vi "MPS_Spectroscopy_Core.vi"(0 "EmptyBoreBaseline_Spec":dbl[](array[numeric])=array[21000 elements], 1 "ms delay":u32=25 format="%#.4p", 3 "Spec samples\nto crop":dbl=1000.0 format="%#_4p") -> (5 "Raw Measured":dbl[](array[numeric]), 6 "f0 Complex":cdb=-0.004151438219837607-0.0046789149193528995i, 7 "phase f1-f9":dbl[](array[numeric])=[-2.296530890286755, -0.4996795442572583, 2.13231335701235, -2.8305146270300687, -3.0644603787657894, -1.910517808964867, -1.4604887262767599, -1.4608770943170013, -0.49288277337997893] format="%#_4g", 8 "TF Corr Rx FFT complex":T2, 9 "TF units from loaded file":string, 10 "Spec Waveform Baseline Sub":waveform(dbl)={"t0"=timestamp(3728232981.5205336 s since 1904-01-01), "dt"=9.9999999999997e-07, "Y"=array[20000 elements], "attributes"=variant("NI_ChannelName"=variant(string "H1/ai7"), "NI_UnitDescription"=variant(string "Volts"))}, 11 "TxIMon cluster":T1, 12 "3f0 Complex":cdb=-1.808865307320394e-10+2.875482942470047e-10i, 13 "mag f1-f9":dbl[](array[numeric])=[0.006255132621749245, 5.349180742819057e-10, 3.3971158138137566e-10, 2.020645150662673e-11, 3.443682420408273e-11, 3.747219651257019e-11, 4.2635827797213496e-11, 3.5893791114801e-11, 3.560739858812373e-11] format="%#_4p", 14 "RX magnitude 3":dbl=3.3971158138137566e-10, 15 "Expected mT Spec Drive":dbl=0.03824103018872398 format="%#_4p", 16 "TF Corrected\nMagnetization over time":waveform(dbl)[](graph), 17 "Spec Time Domain":dbl[][](graph), 18 "Amps Drive Spec":dbl=0.058832354136498434 format="%#_4p", 19 "THD":dbl=1.5484776612982656 format="%#_6p")   [LabVIEW 2021]
uses:
  <vilib>/Analysis/4window.llb/windowTd.ctl
  <extravilib>/ChannelInstances/Tag-dbl/Write With Abort.vi
  MPS_global_variables.vi
  <extravilib>/ChannelInstances/Tag-dbl/Instantiate.vi
  <extravilib>/ChannelInstances/Tag-dbl/Endpoint.vi
  <extravilib>/ChannelInstances/Tag-dbl.lvlib
  <vilib>/measure/NI_MAPro.lvlib
  <vilib>/Analysis/NI_AALPro.lvlib
  <vilib>/measure/matone.llb/Extract Single Tone Information 1 Chan.vi
  <vilib>/measure/maspectr.llb/FFT Spectrum (Mag-Phase) for 1 Chan.vi
panel:
  out "error?":bool
  out "error out":errorcluster
  out "THD dB":dbl
  out "Rx FFT _NoCorrect":cluster{"f0":dbl, "df":dbl, "magnitude":dbl[]}(graph)
  out "f0 over time 2":dbl(graph)=3.3971158138137566e-10
  out "Waveform Graph":cluster{"f0":dbl, "df":dbl, "magnitude":dbl[]}(graph)
  out "dMdt":dbl[](graph)
  out "3f0 over time":dbl(graph)=3.3971158138137566e-10
  out "Drive IMon FFT":cluster{"f0":dbl, "df":dbl, "magnitude":dbl[]}(graph)={"f0"=0.0, "df"=47.61904761904904, "magnitude"=array[10500 elements]}
  out "Drive IMon":waveform(dbl)(graph)={"t0"=timestamp(3728232981.5496345 s since 1904-01-01), "dt"=9.9999999999997e-07, "Y"=array[21000 elements], "attributes"=variant("NI_ChannelName"=variant(string "H1/ai4"), "NI_UnitDescription"=variant(string "Volts"))}
  out "detected amplitude\nDrive IMon":dbl=0.0003328133743989285 format="%.4p"
  out "Samples Per Acquisition":dbl=21000.0
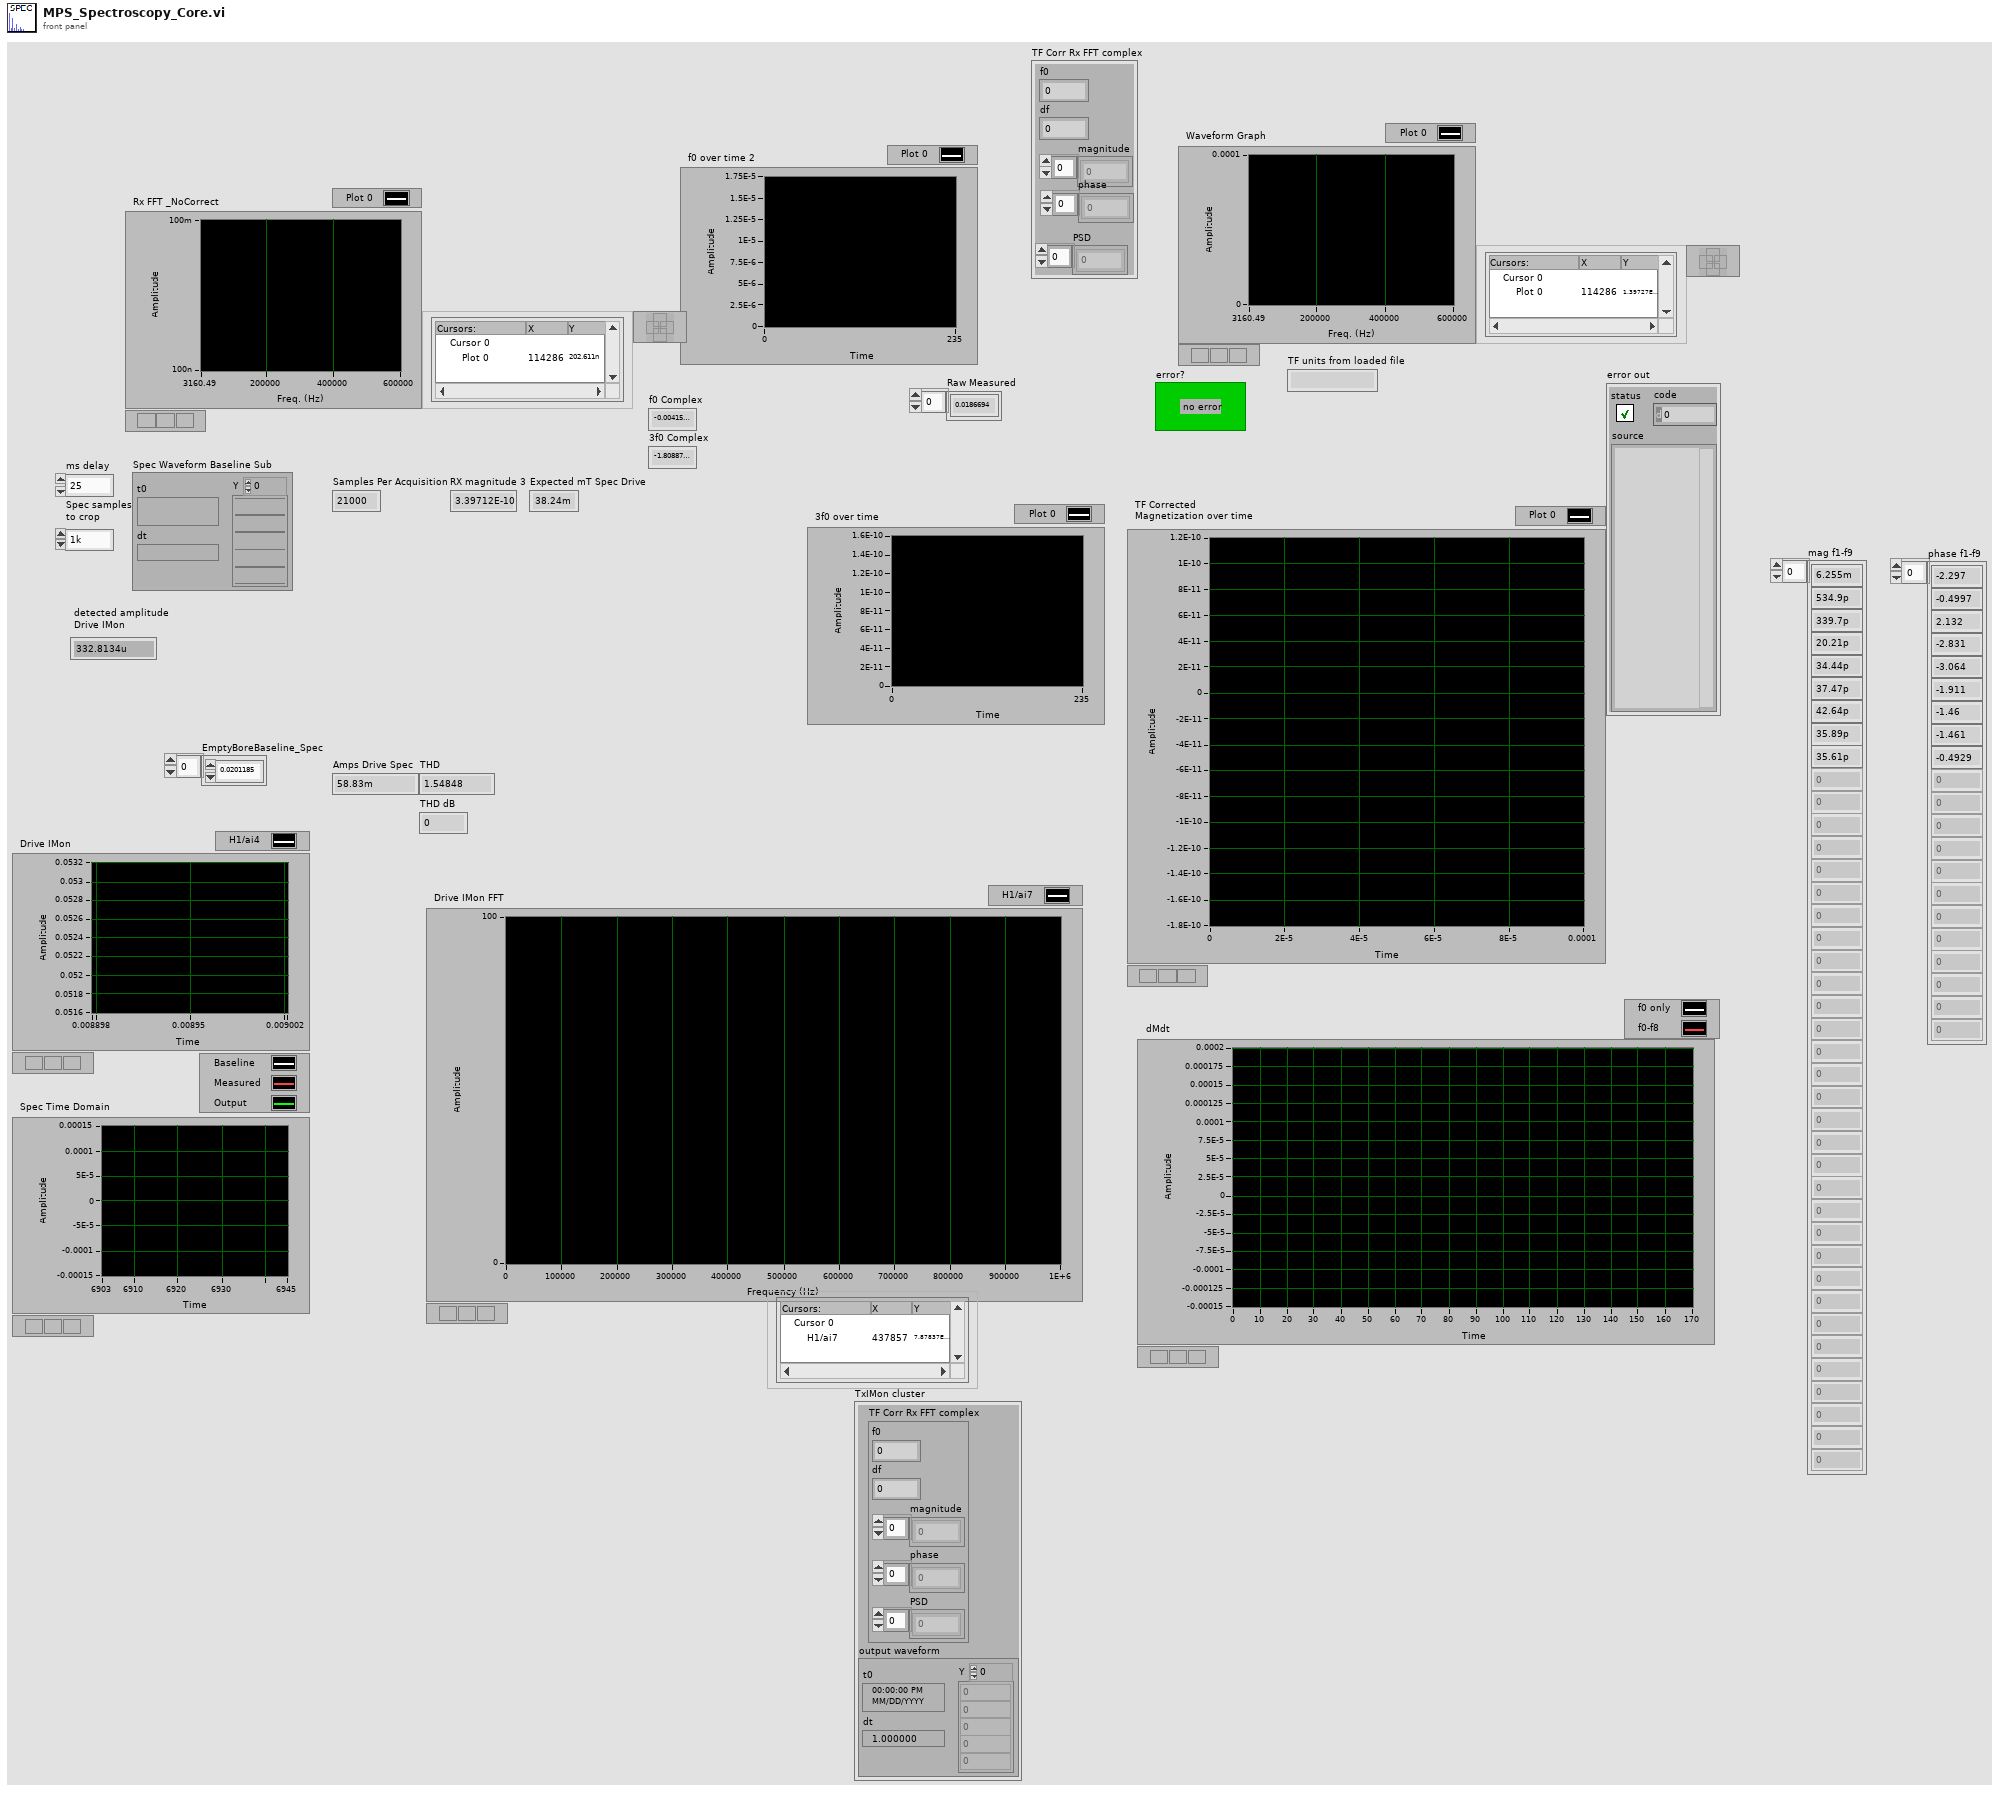
[diagram p1: front panel]
types:
  T1 = cluster{"TF Corr Rx FFT complex":cluster{"f0":dbl, "df":dbl, "magnitude":dbl[], "phase":dbl[], "PSD":dbl[]}, "output waveform":waveform(dbl)}
  T2 = cluster{"f0":dbl, "df":dbl, "magnitude":dbl[], "phase":dbl[], "PSD":dbl[]}
  T3 = cluster{"sample rate":dbl, "Transmit frequency":dbl, "Transmit amplitude":dbl, "sample rate digital out":dbl, "TX cycles":i32, "sample rate DAQ1":dbl, "Receive frequency":dbl, "Receive range":dbl, "TX harmonics":dbl[]}
  T4 = typedef "NI_AALPro.lvlib/windowTd.ctl" = u32
  T5 = cluster{"sample rate":dbl, "Tx freq":dbl, "Tx amp":dbl, "Tx cycles\nSpectroscopy":dbl, "Bias amp":dbl, "Bias freq":dbl, "Receive range":dbl, "Bias Periods\nMagnetometry":dbl, "Tx Freq Division Factor":dbl, "Drive Periods per Bias":dbl, "TX harmonics":dbl[]}
  T6 = typedef "Tag-dbl.lvlib/))Channel.ctl" = refnum<queue>
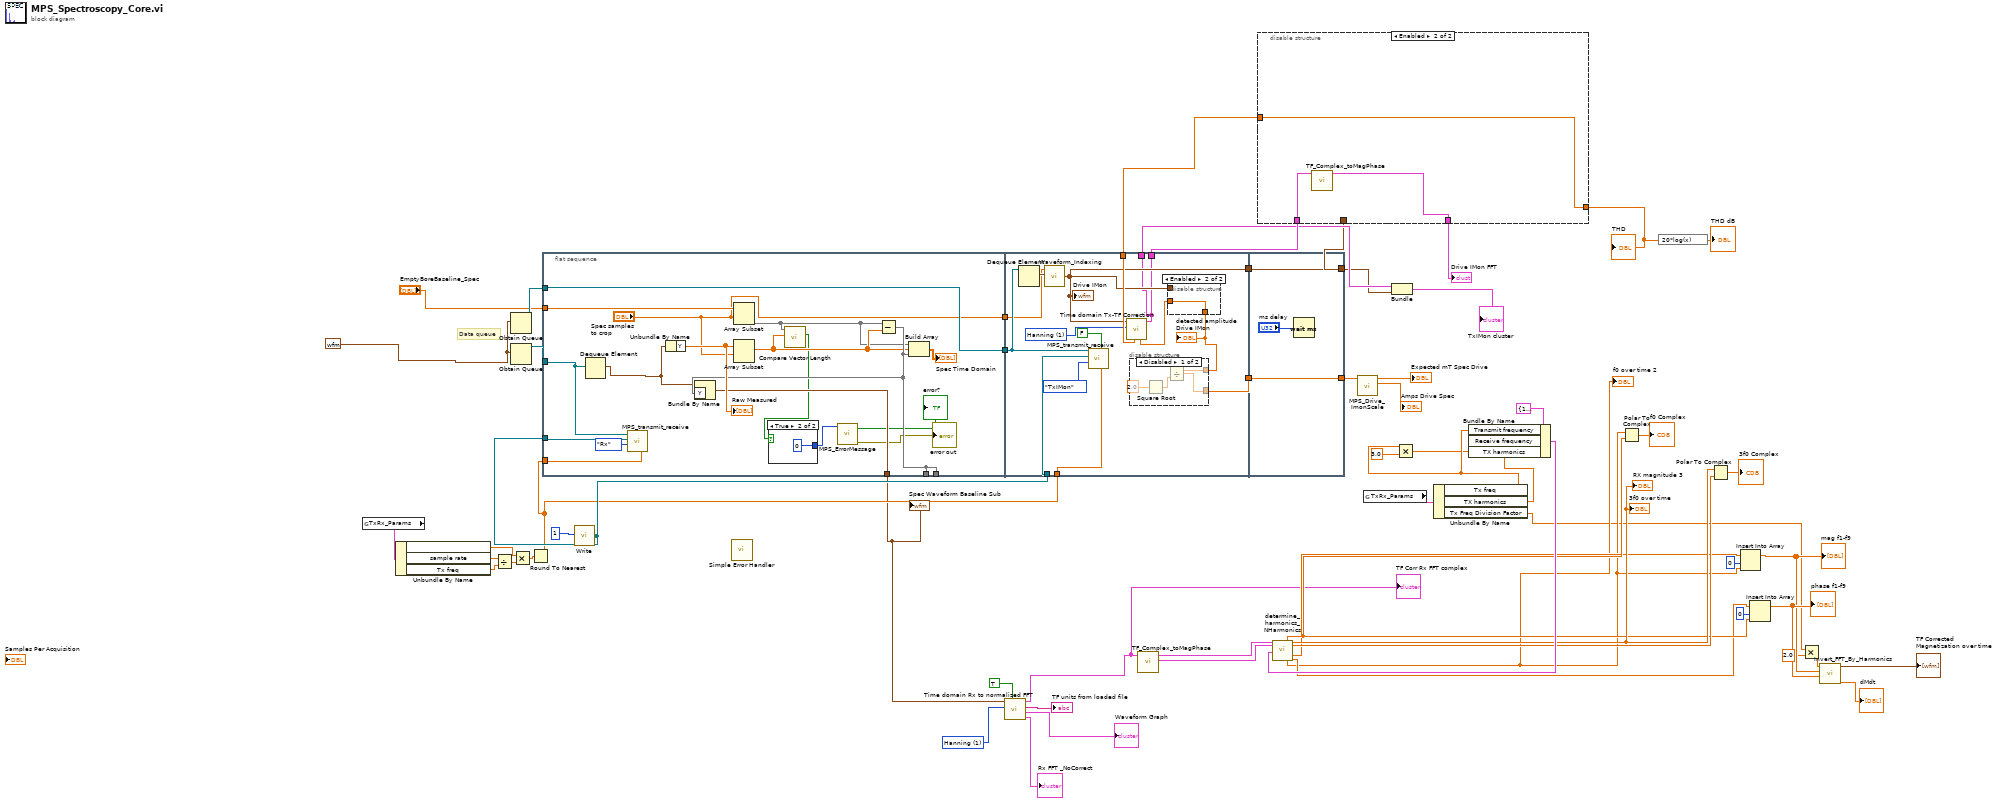
[diagram p0: block diagram]
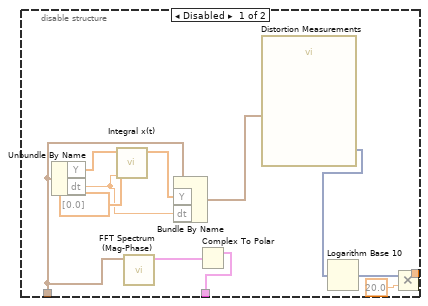
[diagram p2: hidden frame]
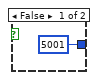
[diagram p3: hidden frame]
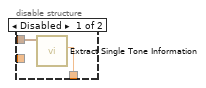
[diagram p5: hidden frame]
diagram:
  w11 = T4 1 items=["Rectangle"=0, "Hanning"=1, "Hamming"=2, "Blackman-Harris"=3, "Exact Blackman"=4, "Blackman"=5, "Flat Top"=6, "4 Term B-Harris "=7, "7 Term B-Harris"=8, "Low Sidelobe"=9, "Blackman Nuttall"=11, "Triangle"=30, "Bartlett-Hanning"=31, "Bohman"=32, "Parzen"=33, "Welch"=34, "Kaiser"=60, "Dolph-Chebyshev"=61, "Gaussian"=62] ("window")
  w23 = waveform(dbl) {"t0"=timestamp(0 s since 1904-01-01), "dt"=1.0, "Y"=[]} ("Waveform")
  # "Data queue"
  n1 = global read "MPS_global_variables.vi" "TxRx_Params"() -> (w54:T5)
  n2 = Unbundle By Name(w54) -> ("Tx cycles\nSpectroscopy"=w50:dbl, "sample rate"=w53:dbl, "Tx freq"=w52:dbl)
  n3 = Divide(x=w53, y=w52) -> (x/y=w51:dbl)
  n4 = Obtain Queue(element data type=w23) -> (queue out=w55:refnum<queue>)  [unwired: 4 in, 2 out]
  n5 = Obtain Queue(element data type=w23) -> (queue out=w56:refnum<queue>)  [unwired: 4 in, 2 out]
  n6 = Multiply(x=w50, y=w51) -> (x*y=w49:dbl)
  n7 = Round To Nearest(number=w49) -> (nearest integer value=w48:dbl)
  n8 = flat-sequence {
    tunnel: w56 -> [w78]
    tunnel: [w77] -> w61
    tunnel: w57 -> [w79]
    tunnel: w55 -> [w77]
    tunnel: w48 -> [w76]
    tunnel: [w73] -> w18
    tunnel: [w72] -> _
    tunnel: [w72] -> _
    tunnel: "EmptyBoreBaseline_Spec" -> [w71]
    tunnel: ["Spec samples\nto crop"] -> w7
    tunnel: w61 -> [w93]
    tunnel: w57 -> [w95]
    tunnel: w48 -> [w94]
    tunnel: [w84] -> w60
    tunnel: [w89] -> w59
    tunnel: [w83] -> w9
    tunnel: [w87] -> w8
    tunnel: w7 -> [w85]
    tunnel: [w83] -> w6
    tunnel: [w106] -> w5
    tunnel: w60 -> [w106]
    tunnel: w59 -> [w104]
    tunnel: [w104] -> w39
    frame #0 {
      n9 = Dequeue Element(queue=w78) -> (element=w69:waveform(dbl))  [unwired: 2 in, 3 out]
      n10 = call "MPS_transmit_receive.vi"("samples per readout"=w76, "InputChans"=enum16{"Rx", "BiasIMon", "TxIMon", "BMon"}."Rx", "channel input for max readouts"=w79, "Measurement Queue"=w78) -> ()  [unwired: 8 in]
      n11 = Unbundle By Name(w69) -> ("Y"=w74:dbl[])
      "Raw Measured" <- w74
      n12 = Array Subset(array=w71, index="Spec samples\nto crop") -> (w66:dbl[])  [unwired: 1 in]
      n13 = Array Subset(array=w74, index="Spec samples\nto crop") -> (w67:dbl[])  [unwired: 1 in]
      n14 = call "Compare Vector Length.vi"("Vec 2"=w67, "Vec 1"=w66) -> ("Length(1) >= Length (2)"=w65:bool)  [unwired: 9 in]
      n15 = case shown="True" w65 {
        tunnel: [5001 ("error code (no error:0)") 0 ("error code (no error:0)")] -> w64
        frame False {
        }
        frame True {
        }
      }
      n16 = call "MPS_ErrorMessage.vi"("error code (no error:0)"=w64) -> ("error out"=→"error out":errorcluster, "error?"=→"error?":bool)  [unwired: 7 in, 2 out]
      n17 = Subtract(x=w66, y=w67) -> (x-y=w72:dbl[])
      n18 = Bundle By Name(cluster=w69, "Y"=w72) -> (w73:waveform(dbl))
      n19 = Build Array(w66, w67, w72) -> (→"Spec Time Domain":dbl[][])
    }
    frame #1 {
      w82 = T4 1 items=["Rectangle"=0, "Hanning"=1, "Hamming"=2, "Blackman-Harris"=3, "Exact Blackman"=4, "Blackman"=5, "Flat Top"=6, "4 Term B-Harris "=7, "7 Term B-Harris"=8, "Low Sidelobe"=9, "Blackman Nuttall"=11, "Triangle"=30, "Bartlett-Hanning"=31, "Bohman"=32, "Parzen"=33, "Welch"=34, "Kaiser"=60, "Dolph-Chebyshev"=61, "Gaussian"=62] ("window")
      n20 = Dequeue Element(queue=w93) -> (element=w86:waveform(dbl))  [unwired: 2 in, 3 out]
      n21 = call "Waveform_Indexing.vi"("index"=w85, "waveform"=w86) -> ("output waveform"=w84:waveform(dbl))  [unwired: 7 in]
      "Drive IMon" <- w84
      n22 = call "MPS_transmit_receive.vi"("samples per readout"=w94, "Use Bias?"=FALSE, "InputChans"=enum16{"Rx", "BiasIMon", "TxIMon", "BMon"}."TxIMon", "channel input for max readouts"=w95, "Measurement Queue"=w93) -> ()  [unwired: 7 in]
      n23 = call "Time domain Tx-TF Correction.vi"("window"=w82, "Tx Waveform"=w84) -> ("TF Corr Rx FFT complex"=w83:T2, "IMon magnitude"=w88:dbl, "THD"=w87:dbl)  [unwired: 4 in, 3 out]
      n24 = disable-structure shown="Enabled" {
        disable-tunnel: [w102 w103] -> w90
        disable-tunnel: w84 -> [w101 _]
        disable-tunnel: w88 -> [_ w103]
        frame Disabled {
          n25 = call-poly <vilib>:"Extract Single Tone Information.vi"("time signal in"=w101) -> ("detected amplitude"=w102:dbl)  [unwired: 5 in, 5 out]
        }
        frame Enabled {
        }
      }
      "detected amplitude\nDrive IMon" <- w90
      n26 = disable-structure shown="Disabled" {
        disable-tunnel: w90 -> [w98 w100]
        disable-tunnel: [w96 w100] -> w89
        frame Disabled {
          n27 = Square Root(x=2.0) -> (sqrt(x)=w99:dbl)
          n28 = Divide(x=w98, y=w99) -> (x/y=w96:dbl)
        }
        frame Enabled {
        }
      }
    }
    frame #2 {
      n29 = Wait (ms)(milliseconds to wait="ms delay") -> ()  [unwired: 1 out]
    }
  }
  n30 = call <extravilib>:"Write.vi"("element"=1 ("number of readouts")) -> ("channel"=w57:T6)  [unwired: 1 out]
  n31 = call <vilib>:"Simple Error Handler.vi"() -> ()  [unwired: 5 in, 5 out]
  n32 = call "Time domain Rx to normalized FFT.vi"("Normalize to TF"=TRUE, "window"=w11, "Spec Waveform Baseline Sub"=w18) -> ("Rx FFT _NoCorrect"=→"Rx FFT _NoCorrect":cluster{"f0":dbl, "df":dbl, "magnitude":dbl[]}, "Waveform Graph"=→"Waveform Graph":cluster{"f0":dbl, "df":dbl, "magnitude":dbl[]}, "TF units from loaded file"=→"TF units from loaded file":string, "TF Corr Rx FFT complex"=w14:T2)  [unwired: 5 in]
  "TF Corr Rx FFT complex" <- w14
  n33 = call "TF_Complex_toMagPhase.vi"("TF Corr Rx FFT Mag"=w14) -> ("TF Phase"=w15:cluster{"f0":dbl, "df":dbl, "magnitude":dbl[]}, "TF Mag"=w16:cluster{"f0":dbl, "df":dbl, "magnitude":dbl[]})  [unwired: 4 in, 5 out]
  n34 = disable-structure shown="Enabled" {
    disable-tunnel: [w115 w119] -> w3
    disable-tunnel: w5 -> [w108 _]
    disable-tunnel: [w107 w120] -> w10
    disable-tunnel: w9 -> [_ w121]
    disable-tunnel: w8 -> [_ w119]
    frame Disabled {
      n35 = Unbundle By Name(w108) -> ("Y"=w114:dbl[], "dt"=w112:dbl)
      n36 = call <vilib>:"Integral x(t).vi"("dt"=w112, "Initial Condition"=dbl[] [0.0], "X"=w114) -> ("Integral X"=w111:dbl[])  [unwired: 7 in, 1 out]
      n37 = call-poly <vilib>:"FFT Spectrum (Mag-Phase).vi"("time signal"=w108) -> ("magnitude"=w109:cluster{"f0":dbl, "df":dbl, "magnitude":dbl[]})  [unwired: 6 in, 4 out]
      n38 = Bundle By Name(cluster=w108, "Y"=w111, "dt"=w112) -> (w110:waveform(dbl))
      n39 = Complex To Polar(r * e^(i*theta)=w109) -> (r=w107:cluster{"f0":dbl, "df":dbl, "magnitude":dbl[]})  [unwired: 1 out]
      n40 = call "Distortion Measurements"("Signals"=w110) -> ("THD"=w118:dynamicdata)  [unwired: 8 in, 2 out]
      n41 = Logarithm Base 10(1:w118) -> (0:w116:dynamicdata)
      n42 = Multiply(x=w116, y=20.0) -> (x*y=w115:dynamicdata)
    }
    frame Enabled {
      n43 = call "TF_Complex_toMagPhase.vi"("TF Corr Rx FFT Mag"=w121) -> ("TF Mag"=w120:cluster{"f0":dbl, "df":dbl, "magnitude":dbl[]})  [unwired: 4 in, 6 out]
    }
  }
  "Drive IMon FFT" <- w10
  "THD" <- w3
  n44 = call "MPS_Drive_ImonScale.vi"("Drive IMon FFT Mag RMS"=w39) -> ("Amps Drive Peak"=→"Amps Drive Spec":dbl, "Expected mT Peak"=→"Expected mT Spec Drive":dbl)  [unwired: 9 in]
  n45 = global read "MPS_global_variables.vi" "TxRx_Params"() -> (w46:T5)
  n46 = Bundle("TF Corr Rx FFT complex"=w6, "output waveform"=w5) -> (→"TxIMon cluster":T1)  [unwired: 1 in]
  n47 = Unbundle By Name(w46) -> ("Tx freq"=w41:dbl, "TX harmonics"=w38:dbl[], "Tx Freq Division Factor"=w19:dbl)
  n48 = Multiply(x=w41, y=3.0) -> (x*y=w40:dbl)
  n49 = Bundle By Name(cluster=T3 {"sample rate"=1000000.0, "Transmit frequency"=25000.0, "Transmit amplitude"=1.577, "sample rate digital out"=40000.0, "TX cycles"=600, "sample rate DAQ1"=1000000.0, "Receive frequency"=75000.0, "Receive range"=1.0, "TX harmonics"=[50000.0, 75000.0, 100000.0, 125000.0, 150000.0, 175000.0, 200000.0, 225000.0]} ("TxRxParams"), "Transmit frequency"=w41, "Receive frequency"=w40, "TX harmonics"=w38) -> (w45:T3)
  n50 = call "determine_harmonics_NHarmonics.vi"("FFT magnitude"=w16, "FFT phase"=w15, "TxRxParams"=w45) -> ("f0 phase"=w30:dbl, "f0 mag"=w22:dbl, "RX magnitude"=w34:dbl, "RX phase"=w35:dbl, "mag 2f0-Nf0"=w28:dbl[], "phase 2f0-Nf0"=w29:dbl[])  [unwired: 11 in]
  "RX magnitude 3" <- w34
  "3f0 over time" <- w34
  "f0 over time 2" <- w22
  n51 = Polar To Complex(1:w30, 2:w22) -> (0:→"f0 Complex":cdb)
  n52 = expression code="20*log(x)"(w3) -> (→"THD dB":dbl)
  n53 = Polar To Complex(1:w35, 2:w34) -> (0:→"3f0 Complex":cdb)
  n54 = Insert Into Array(array=w28, index=0, new element=w22) -> (w25:dbl[])
  "mag f1-f9" <- w25
  n55 = Insert Into Array(array=w29, index=0, new element=w30) -> (w26:dbl[])
  "phase f1-f9" <- w26
  n56 = Multiply(x=w19, y=2.0) -> (x*y=w21:dbl)
  n57 = call "Invert_FFT_By_Harmonics.vi"("phase f1-f9"=w26, "mag f1-f9"=w25, "Num Samp"=w21) -> ("dMdt"=→"dMdt":dbl[], "Waveform Graph"=→"TF Corrected\nMagnetization over time":waveform(dbl)[])  [unwired: 6 in, 1 out]
  "Spec Waveform Baseline Sub" <- w18
